vi "Hitrap_DiagnosticBoxGUI.get status.vi"(1 "DIMArray":refnum<notifier>[](array[refnum]), 2 "NofAxes":i32, 3 "Axis":i32, 5 "error in (no error)":errorcluster) -> (10 "deviceState":i32, 11 "Reference":bool=TRUE, 12 "Error":bool=TRUE, 13 "Enable":bool=TRUE, 14 "AutoHalt?":bool, 15 "actValueStatu":T1 items=["motorEnabled"=1, "negativeLimitSwitchActive"=2, "positiveLimitSwitchActive"=4, "limitSwitchesEnabled"=8, "limitSwitchesAreNormallyClosed"=16, "moving"=32, "referenced"=64, "inPosition"=128, "reserved2"=256, "reserved3"=512, "reserved4"=1024, "reserved5"=2048, "error"=4096, "reserved6"=8192, "reserved7"=16384, "reserved8"=32768, "user defined1"=65536, "user defined2"=131072, "user defined3"=262144, "user defined4"=524288, "user defined5"=1048576, "user defined6"=2097152, "user defined7"=4194304, "user defined8"=8388608, "user defined9"=16777216, "user defined10"=33554432, "user defined11"=67108864, "user defined12"=134217728, "user defined13"=268435456, "user defined14"=536870912, "user defined15"=1073741824, "user defined16"=2147483648], 16 "Position":dbl, 17 "Moving":bool=TRUE, 18 "in Position":bool=TRUE, 19 "error out":errorcluster)   [LabVIEW 2014, in "Hitrap_DiagnosticBoxGUI.lvlib"]
doc: "obtain the actual status of the device (from the class motor base)."
uses:
  Hitrap_DiagnosticBoxGUI.lvlib
  CSCore/CSApplicationBaseClasses/MotorBase/MotorBase.statusType.ctl
  CSCore/CSApplicationBaseClasses/MotorBase/MotorBase.lvlib
  CSlibraries-extern/DimLVEvent/LVDimInterface/LVDimInterface.lvlib
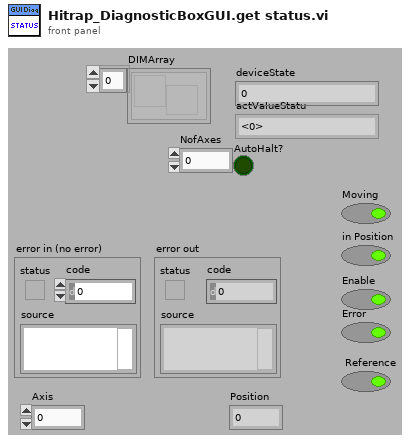
[diagram p1: front panel]
types:
  T1 = typedef "MotorBase.lvlib/MotorBase.statusType.ctl" = u32
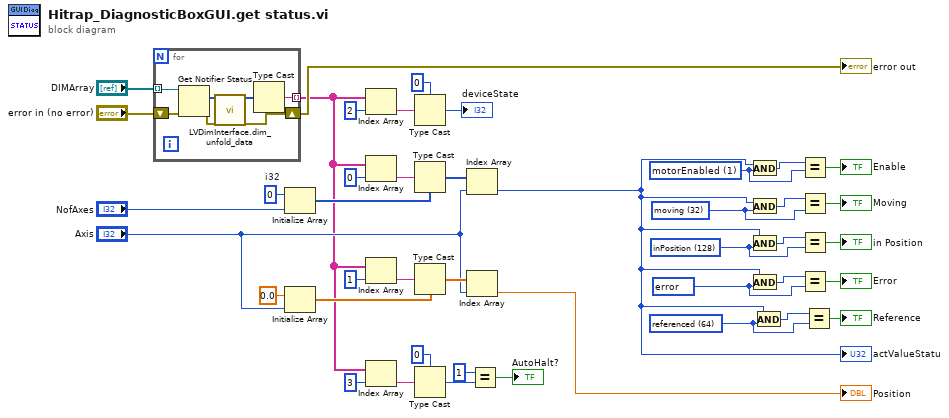
[diagram p0: block diagram]
diagram:
  w28 = 0  # i32
  w29 = T1 64 items=["motorEnabled"=1, "negativeLimitSwitchActive"=2, "positiveLimitSwitchActive"=4, "limitSwitchesEnabled"=8, "limitSwitchesAreNormallyClosed"=16, "moving"=32, "referenced"=64, "inPosition"=128, "reserved2"=256, "reserved3"=512, "reserved4"=1024, "reserved5"=2048, "error"=4096, "reserved6"=8192, "reserved7"=16384, "reserved8"=32768, "user defined1"=65536, "user defined2"=131072, "user defined3"=262144, "user defined4"=524288, "user defined5"=1048576, "user defined6"=2097152, "user defined7"=4194304, "user defined8"=8388608, "user defined9"=16777216, "user defined10"=33554432, "user defined11"=67108864, "user defined12"=134217728, "user defined13"=268435456, "user defined14"=536870912, "user defined15"=1073741824, "user defined16"=2147483648] ("y")
  w31 = T1 4096 items=["motorEnabled"=1, "negativeLimitSwitchActive"=2, "positiveLimitSwitchActive"=4, "limitSwitchesEnabled"=8, "limitSwitchesAreNormallyClosed"=16, "moving"=32, "referenced"=64, "inPosition"=128, "reserved2"=256, "reserved3"=512, "reserved4"=1024, "reserved5"=2048, "error"=4096, "reserved6"=8192, "reserved7"=16384, "reserved8"=32768, "user defined1"=65536, "user defined2"=131072, "user defined3"=262144, "user defined4"=524288, "user defined5"=1048576, "user defined6"=2097152, "user defined7"=4194304, "user defined8"=8388608, "user defined9"=16777216, "user defined10"=33554432, "user defined11"=67108864, "user defined12"=134217728, "user defined13"=268435456, "user defined14"=536870912, "user defined15"=1073741824, "user defined16"=2147483648] ("y")
  w36 = T1 1 items=["motorEnabled"=1, "negativeLimitSwitchActive"=2, "positiveLimitSwitchActive"=4, "limitSwitchesEnabled"=8, "limitSwitchesAreNormallyClosed"=16, "moving"=32, "referenced"=64, "inPosition"=128, "reserved2"=256, "reserved3"=512, "reserved4"=1024, "reserved5"=2048, "error"=4096, "reserved6"=8192, "reserved7"=16384, "reserved8"=32768, "user defined1"=65536, "user defined2"=131072, "user defined3"=262144, "user defined4"=524288, "user defined5"=1048576, "user defined6"=2097152, "user defined7"=4194304, "user defined8"=8388608, "user defined9"=16777216, "user defined10"=33554432, "user defined11"=67108864, "user defined12"=134217728, "user defined13"=268435456, "user defined14"=536870912, "user defined15"=1073741824, "user defined16"=2147483648] ("y")
  w38 = T1 32 items=["motorEnabled"=1, "negativeLimitSwitchActive"=2, "positiveLimitSwitchActive"=4, "limitSwitchesEnabled"=8, "limitSwitchesAreNormallyClosed"=16, "moving"=32, "referenced"=64, "inPosition"=128, "reserved2"=256, "reserved3"=512, "reserved4"=1024, "reserved5"=2048, "error"=4096, "reserved6"=8192, "reserved7"=16384, "reserved8"=32768, "user defined1"=65536, "user defined2"=131072, "user defined3"=262144, "user defined4"=524288, "user defined5"=1048576, "user defined6"=2097152, "user defined7"=4194304, "user defined8"=8388608, "user defined9"=16777216, "user defined10"=33554432, "user defined11"=67108864, "user defined12"=134217728, "user defined13"=268435456, "user defined14"=536870912, "user defined15"=1073741824, "user defined16"=2147483648] ("y")
  w34 = T1 128 items=["motorEnabled"=1, "negativeLimitSwitchActive"=2, "positiveLimitSwitchActive"=4, "limitSwitchesEnabled"=8, "limitSwitchesAreNormallyClosed"=16, "moving"=32, "referenced"=64, "inPosition"=128, "reserved2"=256, "reserved3"=512, "reserved4"=1024, "reserved5"=2048, "error"=4096, "reserved6"=8192, "reserved7"=16384, "reserved8"=32768, "user defined1"=65536, "user defined2"=131072, "user defined3"=262144, "user defined4"=524288, "user defined5"=1048576, "user defined6"=2097152, "user defined7"=4194304, "user defined8"=8388608, "user defined9"=16777216, "user defined10"=33554432, "user defined11"=67108864, "user defined12"=134217728, "user defined13"=268435456, "user defined14"=536870912, "user defined15"=1073741824, "user defined16"=2147483648] ("y")
  n1 = for {
    tunnel: "DIMArray" -> [w48] mode=indexing
    tunnel: [w47] -> w4 mode=indexing
    shift-right: [w44] -> w8
    shift-left: "error in (no error)" -> [w46]
    n2 = Get Notifier Status(notifier=w48, error in (no error)=w46) -> (current notification=w49:i8[], error out=w45:errorcluster)  [unwired: 3 out]
    n3 = call "LVDimInterface.dim_unfold_data.vi"("rawData"=w49, "error in (no error)"=w45) -> ("data"=w50:i8[], "error out"=w44:errorcluster)  [unwired: 14 in, 2 out]
    n4 = Type Cast(x=w50) -> (*(type *) &x=w47:string)  [unwired: 1 in]
  }
  "error out" <- w8
  n5 = Initialize Array(w28, "NofAxes") -> (w19:i32[])
  n6 = Initialize Array(0.0, "Axis") -> (w14:dbl[])
  n7 = Index Array(array=w4, index=2) -> (element=w24:string)
  n8 = Index Array(array=w4, index=0) -> (element=w20:string)
  n9 = Index Array(array=w4, index=1) -> (element=w15:string)
  n10 = Index Array(array=w4, index=3) -> (element=w6:string)
  n11 = Type Cast(type=0 ("index"), x=w24) -> (*(type *) &x=→"deviceState":i32)
  n12 = Type Cast(type=w19, x=w20) -> (*(type *) &x=w18:i32[])
  n13 = Type Cast(type=w14, x=w15) -> (*(type *) &x=w12:dbl[])
  n14 = Type Cast(type=0 ("index"), x=w6) -> (*(type *) &x=w3:i32)
  n15 = Index Array(array=w18, index="Axis") -> (element=w17:i32)
  "actValueStatu" <- w17
  n16 = Index Array(array=w12, index="Axis") -> (element=→"Position":dbl)
  n17 = Equal?(x=1, y=w3) -> (x = y?=→"AutoHalt?":bool)
  n18 = And(x=w17, y=w36) -> (x .and. y?=w37:T1)
  n19 = And(x=w17, y=w38) -> (x .and. y?=w39:T1)
  n20 = And(x=w17, y=w34) -> (x .and. y?=w33:T1)
  n21 = And(x=w17, y=w31) -> (x .and. y?=w32:T1)
  n22 = And(x=w17, y=w29) -> (x .and. y?=w30:T1)
  n23 = Equal?(x=w37, y=w36) -> (x = y?=→"Enable":bool)
  n24 = Equal?(x=w39, y=w38) -> (x = y?=→"Moving":bool)
  n25 = Equal?(x=w33, y=w34) -> (x = y?=→"in Position":bool)
  n26 = Equal?(x=w32, y=w31) -> (x = y?=→"Error":bool)
  n27 = Equal?(x=w30, y=w29) -> (x = y?=→"Reference":bool)
